vi "Defect Inspection.vi"() -> ()   [LabVIEW 2016]
doc: "Demonstrate how to use the IMAQ Calculate Defect Map function to find defects in images."
uses:
  <vilib>/vision/Pattern Matching.llb/IMAQ Pattern Match Advanced Options.ctl
  <vilib>/vision/NI_Vision_Development_Module.lvlib
panel:
  out "Thresholded Defect Map":T1(plugin-control)
  out "Defect Map":T1(plugin-control)
  out "Inspection Image":T1(plugin-control)
  out "Weight Map":T1(plugin-control)
  in  "Select Image":i32(slide) min=0 max=5 step=1 scale=0.0..4.0
  in  "Stop Button":bool
  out "Template":T1(plugin-control)
  # "Overview: Demonstrate how to use the IMAQ Calculate Defect Map function to find defects in images.\nThe VI loads a template with a pre-defined Weight Map and calls IMAQ Match Pattern 4  to find a match. IMAQ Calculate Defect Map calculates the defect map with a score for every pixel. High scores indicate a high probability for the pixels to be a defect.\nRequirements: Vision Development Module.\n\nInstructions:\n1. Run the VI.\n2. Use \"Select Image\" control to process a different image."
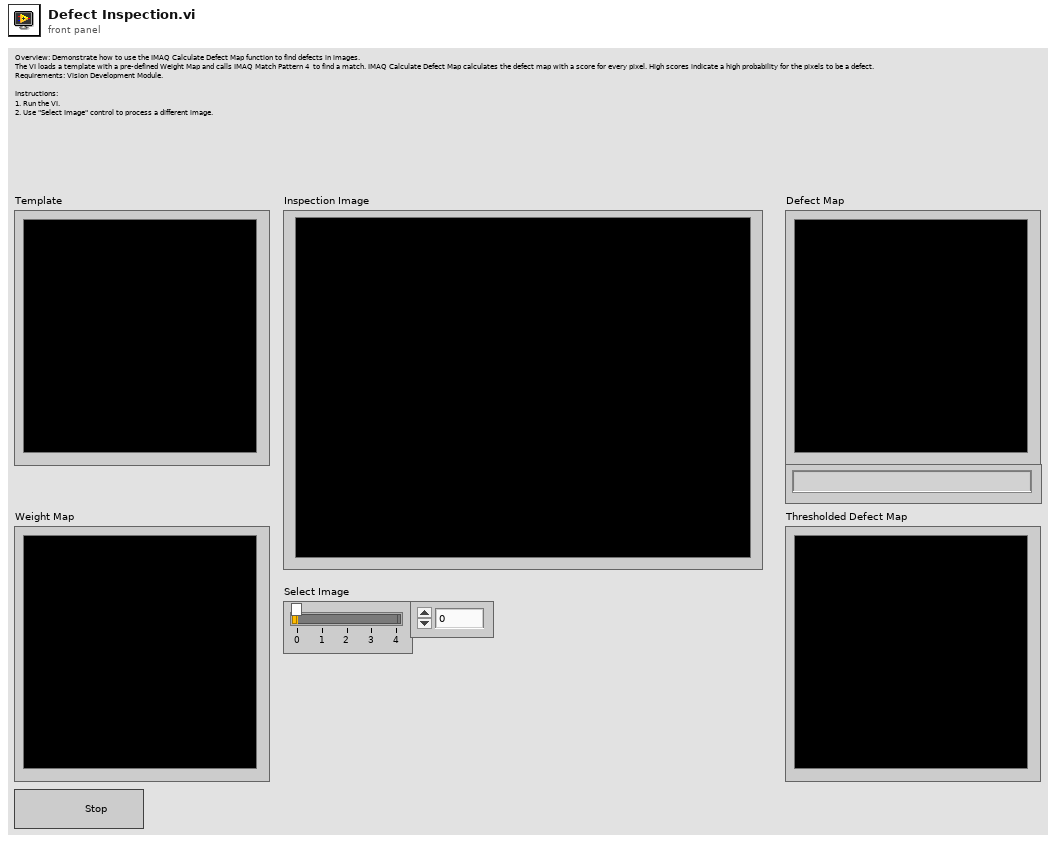
[diagram p1: front panel]
types:
  T1 = typedef "IMAQ Image.ctl" = refnum<image>
  T2 = typedef "Image Type" = u32
  T3 = typedef "IMAQ Pattern Match Advanced Options.ctl" = u16
  T4 = cluster{"Number of Matches Requested":i32, "Minimum Match Score":sgl, "Angle Ranges":cluster{"Start Angle":sgl, "End Angle":sgl}[]}
  T5 = cluster{"Position":cluster{"x":sgl, "y":sgl}, "Angle":sgl, "Scale":sgl, "Score":sgl, "Bounding Box":cluster{"x":sgl, "y":sgl}[]}[]
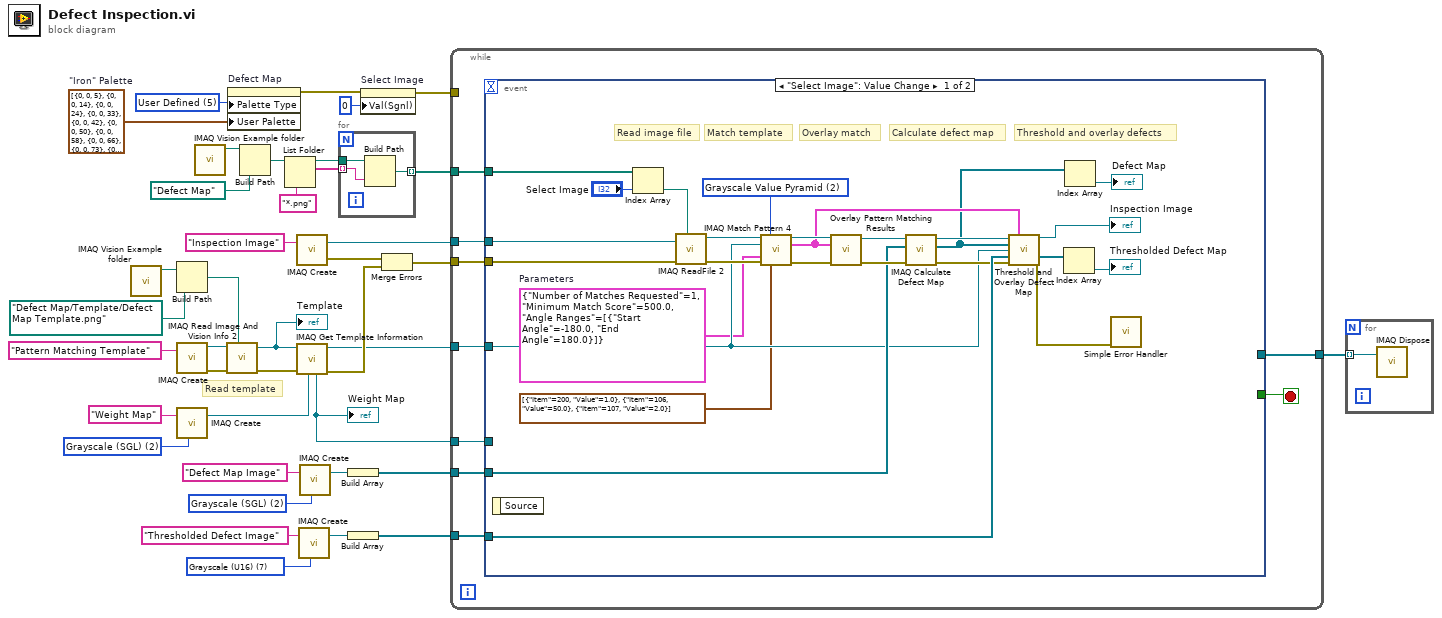
[diagram p0: block diagram]
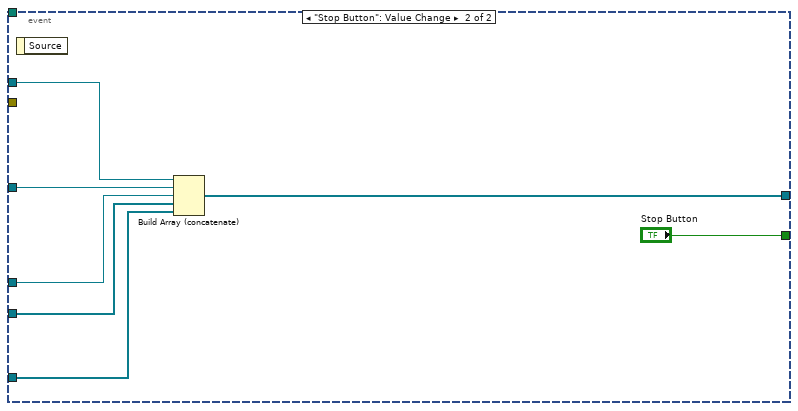
[diagram p2: hidden frame]
diagram:
  w3 = u32 5 items=["Grayscale", "Binary", "Gradient", "Rainbow", "Temperature", "User Defined", "Binary 16 Bit", "Gradient 16 Bit", "Rainbow 16 Bit", "Temperature 16 Bit", "User Defined 16 Bit"] ("Palette:Palette Type")
  w2 = cluster{"Red":u8, "Green":u8, "Blue":u8}[] [{"Red"=0, "Green"=0, "Blue"=5}, {"Red"=0, "Green"=0, "Blue"=14}, {"Red"=0, "Green"=0, "Blue"=24}, {"Red"=0, "Green"=0, "Blue"=33}, {"Red"=0, "Green"=0, "Blue"=42}, {"Red"=0, "Green"=0, "Blue"=50}, {"Red"=0, "Green"=0, "Blue"=58}, {"Red"=0, "Green"=0, "Blue"=66}, {"Red"=0, "Green"=0, "Blue"=73}, {"Red"=0, "Green"=0, "Blue"=80}, {"Red"=0, "Green"=0, "Blue"=86}, {"Red"=0, "Green"=0, "Blue"=91}, {"Red"=1, "Green"=0, "Blue"=96}, {"Red"=2, "Green"=0, "Blue"=100}, {"Red"=3, "Green"=0, "Blue"=103}, {"Red"=4, "Green"=0, "Blue"=106}, {"Red"=5, "Green"=0, "Blue"=109}, {"Red"=7, "Green"=0, "Blue"=111}, {"Red"=9, "Green"=0, "Blue"=114}, {"Red"=11, "Green"=0, "Blue"=116}, {"Red"=13, "Green"=0, "Blue"=118}, {"Red"=16, "Green"=0, "Blue"=120}, {"Red"=18, "Green"=0, "Blue"=122}, {"Red"=21, "Green"=0, "Blue"=125}, {"Red"=24, "Green"=0, "Blue"=127}, {"Red"=28, "Green"=0, "Blue"=129}, {"Red"=31, "Green"=0, "Blue"=131}, {"Red"=34, "Green"=0, "Blue"=133}, {"Red"=38, "Green"=0, "Blue"=135}, {"Red"=41, "Green"=0, "Blue"=137}, {"Red"=44, "Green"=0, "Blue"=139}, {"Red"=47, "Green"=0, "Blue"=141}, {"Red"=50, "Green"=0, "Blue"=142}, {"Red"=53, "Green"=0, "Blue"=144}, {"Red"=56, "Green"=0, "Blue"=145}, {"Red"=59, "Green"=0, "Blue"=146}, {"Red"=61, "Green"=0, "Blue"=147}, {"Red"=64, "Green"=0, "Blue"=149}, {"Red"=67, "Green"=0, "Blue"=149}, {"Red"=69, "Green"=0, "Blue"=150}, {"Red"=72, "Green"=0, "Blue"=151}, {"Red"=75, "Green"=0, "Blue"=152}, {"Red"=77, "Green"=0, "Blue"=152}, {"Red"=80, "Green"=0, "Blue"=153}, {"Red"=83, "Green"=0, "Blue"=153}, {"Red"=86, "Green"=0, "Blue"=154}, {"Red"=89, "Green"=0, "Blue"=154}, {"Red"=91, "Green"=0, "Blue"=154}, {"Red"=94, "Green"=0, "Blue"=154}, {"Red"=97, "Green"=0, "Blue"=155}, {"Red"=100, "Green"=0, "Blue"=155}, {"Red"=103, "Green"=0, "Blue"=155}, {"Red"=106, "Green"=0, "Blue"=156}, {"Red"=109, "Green"=0, "Blue"=156}, {"Red"=112, "Green"=0, "Blue"=156}, {"Red"=115, "Green"=0, "Blue"=156}, {"Red"=117, "Green"=0, "Blue"=157}, {"Red"=120, "Green"=0, "Blue"=157}, {"Red"=123, "Green"=0, "Blue"=157}, {"Red"=126, "Green"=0, "Blue"=157}, {"Red"=129, "Green"=0, "Blue"=157}, {"Red"=132, "Green"=0, "Blue"=157}, {"Red"=135, "Green"=0, "Blue"=157}, {"Red"=137, "Green"=0, "Blue"=157}, {"Red"=140, "Green"=0, "Blue"=157}, {"Red"=143, "Green"=0, "Blue"=156}, {"Red"=146, "Green"=0, "Blue"=156}, {"Red"=148, "Green"=0, "Blue"=156}, {"Red"=151, "Green"=0, "Blue"=156}, {"Red"=154, "Green"=0, "Blue"=155}, {"Red"=156, "Green"=0, "Blue"=155}, {"Red"=158, "Green"=0, "Blue"=155}, {"Red"=161, "Green"=0, "Blue"=154}, {"Red"=163, "Green"=0, "Blue"=154}, {"Red"=165, "Green"=0, "Blue"=154}, {"Red"=167, "Green"=0, "Blue"=153}, {"Red"=170, "Green"=0, "Blue"=153}, {"Red"=172, "Green"=0, "Blue"=152}, {"Red"=173, "Green"=0, "Blue"=152}, {"Red"=175, "Green"=0, "Blue"=152}, {"Red"=177, "Green"=0, "Blue"=151}, {"Red"=179, "Green"=0, "Blue"=150}, {"Red"=180, "Green"=1, "Blue"=150}, {"Red"=182, "Green"=1, "Blue"=149}, {"Red"=183, "Green"=2, "Blue"=148}, {"Red"=185, "Green"=2, "Blue"=148}, {"Red"=186, "Green"=3, "Blue"=147}, {"Red"=187, "Green"=4, "Blue"=146}, {"Red"=188, "Green"=4, "Blue"=146}, {"Red"=190, "Green"=5, "Blue"=145}, {"Red"=191, "Green"=6, "Blue"=144}, {"Red"=192, "Green"=7, "Blue"=143}, {"Red"=194, "Green"=8, "Blue"=142}, {"Red"=195, "Green"=9, "Blue"=142}, {"Red"=196, "Green"=10, "Blue"=141}, {"Red"=197, "Green"=11, "Blue"=140}, {"Red"=198, "Green"=13, "Blue"=139}, {"Red"=200, "Green"=14, "Blue"=137}, {"Red"=201, "Green"=15, "Blue"=136}, {"Red"=202, "Green"=17, "Blue"=135}, {"Red"=203, "Green"=18, "Blue"=133}, {"Red"=204, "Green"=20, "Blue"=131}, {"Red"=205, "Green"=21, "Blue"=129}, {"Red"=206, "Green"=23, "Blue"=127}, {"Red"=207, "Green"=24, "Blue"=125}, {"Red"=208, "Green"=26, "Blue"=122}, {"Red"=209, "Green"=28, "Blue"=119}, {"Red"=210, "Green"=30, "Blue"=116}, {"Red"=211, "Green"=31, "Blue"=113}, {"Red"=212, "Green"=33, "Blue"=110}, {"Red"=213, "Green"=35, "Blue"=106}, {"Red"=214, "Green"=37, "Blue"=102}, {"Red"=215, "Green"=39, "Blue"=98}, {"Red"=216, "Green"=40, "Blue"=94}, {"Red"=217, "Green"=42, "Blue"=89}, {"Red"=218, "Green"=44, "Blue"=85}, {"Red"=219, "Green"=46, "Blue"=80}, {"Red"=220, "Green"=48, "Blue"=75}, {"Red"=221, "Green"=49, "Blue"=71}, {"Red"=222, "Green"=51, "Blue"=66}, {"Red"=223, "Green"=53, "Blue"=61}, {"Red"=224, "Green"=55, "Blue"=56}, {"Red"=225, "Green"=57, "Blue"=51}, {"Red"=226, "Green"=58, "Blue"=47}, {"Red"=227, "Green"=60, "Blue"=42}, {"Red"=228, "Green"=62, "Blue"=38}, {"Red"=229, "Green"=64, "Blue"=34}, {"Red"=230, "Green"=66, "Blue"=30}, {"Red"=231, "Green"=67, "Blue"=26}, {"Red"=231, "Green"=69, "Blue"=23}, {"Red"=232, "Green"=71, "Blue"=20}, {"Red"=233, "Green"=73, "Blue"=17}, {"Red"=233, "Green"=75, "Blue"=15}, {"Red"=234, "Green"=77, "Blue"=13}, {"Red"=234, "Green"=78, "Blue"=12}, {"Red"=235, "Green"=80, "Blue"=10}, {"Red"=235, "Green"=82, "Blue"=9}, {"Red"=236, "Green"=84, "Blue"=8}, {"Red"=236, "Green"=86, "Blue"=7}, {"Red"=237, "Green"=87, "Blue"=7}, {"Red"=237, "Green"=89, "Blue"=6}, {"Red"=237, "Green"=91, "Blue"=5}, {"Red"=238, "Green"=92, "Blue"=5}, {"Red"=239, "Green"=94, "Blue"=4}, {"Red"=239, "Green"=95, "Blue"=4}, {"Red"=240, "Green"=97, "Blue"=4}, {"Red"=240, "Green"=98, "Blue"=3}, {"Red"=241, "Green"=100, "Blue"=3}, {"Red"=241, "Green"=101, "Blue"=3}, {"Red"=242, "Green"=102, "Blue"=2}, {"Red"=242, "Green"=104, "Blue"=2}, {"Red"=242, "Green"=106, "Blue"=2}, {"Red"=243, "Green"=107, "Blue"=1}, {"Red"=243, "Green"=109, "Blue"=1}, {"Red"=243, "Green"=111, "Blue"=1}, {"Red"=244, "Green"=112, "Blue"=1}, {"Red"=244, "Green"=114, "Blue"=1}, {"Red"=244, "Green"=116, "Blue"=0}, {"Red"=244, "Green"=117, "Blue"=0}, {"Red"=245, "Green"=119, "Blue"=0}, {"Red"=245, "Green"=121, "Blue"=0}, {"Red"=245, "Green"=123, "Blue"=0}, {"Red"=246, "Green"=125, "Blue"=0}, {"Red"=246, "Green"=126, "Blue"=0}, {"Red"=247, "Green"=128, "Blue"=0}, {"Red"=247, "Green"=130, "Blue"=0}, {"Red"=247, "Green"=132, "Blue"=0}, {"Red"=248, "Green"=134, "Blue"=0}, {"Red"=248, "Green"=135, "Blue"=0}, {"Red"=249, "Green"=137, "Blue"=0}, {"Red"=249, "Green"=139, "Blue"=0}, {"Red"=249, "Green"=141, "Blue"=0}, {"Red"=250, "Green"=143, "Blue"=0}, {"Red"=250, "Green"=145, "Blue"=0}, {"Red"=250, "Green"=147, "Blue"=0}, {"Red"=251, "Green"=148, "Blue"=0}, {"Red"=251, "Green"=150, "Blue"=0}, {"Red"=251, "Green"=152, "Blue"=0}, {"Red"=252, "Green"=154, "Blue"=0}, {"Red"=252, "Green"=156, "Blue"=0}, {"Red"=252, "Green"=158, "Blue"=0}, {"Red"=252, "Green"=160, "Blue"=0}, {"Red"=252, "Green"=162, "Blue"=0}, {"Red"=253, "Green"=164, "Blue"=0}, {"Red"=253, "Green"=166, "Blue"=0}, {"Red"=253, "Green"=167, "Blue"=0}, {"Red"=253, "Green"=169, "Blue"=0}, {"Red"=253, "Green"=171, "Blue"=0}, {"Red"=254, "Green"=173, "Blue"=0}, {"Red"=254, "Green"=175, "Blue"=0}, {"Red"=254, "Green"=177, "Blue"=0}, {"Red"=254, "Green"=179, "Blue"=0}, {"Red"=254, "Green"=181, "Blue"=0}, {"Red"=255, "Green"=183, "Blue"=0}, {"Red"=255, "Green"=185, "Blue"=0}, {"Red"=255, "Green"=187, "Blue"=0}, {"Red"=255, "Green"=189, "Blue"=0}, {"Red"=255, "Green"=191, "Blue"=0}, {"Red"=255, "Green"=192, "Blue"=0}, {"Red"=255, "Green"=194, "Blue"=0}, {"Red"=255, "Green"=196, "Blue"=0}, {"Red"=255, "Green"=198, "Blue"=0}, {"Red"=255, "Green"=199, "Blue"=1}, {"Red"=255, "Green"=201, "Blue"=1}, {"Red"=255, "Green"=203, "Blue"=2}, {"Red"=254, "Green"=204, "Blue"=2}, {"Red"=254, "Green"=206, "Blue"=3}, {"Red"=254, "Green"=208, "Blue"=4}, {"Red"=254, "Green"=209, "Blue"=5}, {"Red"=254, "Green"=211, "Blue"=7}, {"Red"=254, "Green"=212, "Blue"=8}, {"Red"=254, "Green"=213, "Blue"=10}, {"Red"=254, "Green"=215, "Blue"=11}, {"Red"=254, "Green"=216, "Blue"=13}, {"Red"=254, "Green"=218, "Blue"=15}, {"Red"=254, "Green"=219, "Blue"=18}, {"Red"=255, "Green"=221, "Blue"=21}, {"Red"=255, "Green"=222, "Blue"=24}, {"Red"=255, "Green"=223, "Blue"=27}, {"Red"=255, "Green"=225, "Blue"=31}, {"Red"=255, "Green"=226, "Blue"=35}, {"Red"=255, "Green"=227, "Blue"=40}, {"Red"=255, "Green"=229, "Blue"=44}, {"Red"=255, "Green"=230, "Blue"=50}, {"Red"=255, "Green"=231, "Blue"=55}, {"Red"=255, "Green"=233, "Blue"=61}, {"Red"=255, "Green"=234, "Blue"=67}, {"Red"=255, "Green"=235, "Blue"=74}, {"Red"=255, "Green"=236, "Blue"=80}, {"Red"=255, "Green"=237, "Blue"=87}, {"Red"=255, "Green"=238, "Blue"=94}, {"Red"=255, "Green"=239, "Blue"=101}, {"Red"=255, "Green"=240, "Blue"=108}, {"Red"=255, "Green"=240, "Blue"=115}, {"Red"=255, "Green"=241, "Blue"=122}, {"Red"=255, "Green"=242, "Blue"=130}, {"Red"=255, "Green"=243, "Blue"=137}, {"Red"=255, "Green"=243, "Blue"=144}, {"Red"=255, "Green"=244, "Blue"=151}, {"Red"=255, "Green"=244, "Blue"=157}, {"Red"=255, "Green"=245, "Blue"=164}, {"Red"=255, "Green"=246, "Blue"=170}, {"Red"=255, "Green"=246, "Blue"=177}, {"Red"=255, "Green"=247, "Blue"=183}, {"Red"=255, "Green"=248, "Blue"=189}, {"Red"=255, "Green"=248, "Blue"=195}, {"Red"=255, "Green"=249, "Blue"=200}, {"Red"=255, "Green"=250, "Blue"=206}, {"Red"=255, "Green"=251, "Blue"=212}, {"Red"=255, "Green"=251, "Blue"=217}, {"Red"=255, "Green"=252, "Blue"=223}, {"Red"=255, "Green"=253, "Blue"=229}, {"Red"=255, "Green"=253, "Blue"=234}, {"Red"=255, "Green"=254, "Blue"=240}, {"Red"=255, "Green"=255, "Blue"=246}, {"Red"=255, "Green"=255, "Blue"=251}]  # "Iron" Palette
  w11 = T2 7 items=["Grayscale (U8)", "Grayscale (I16)", "Grayscale (SGL)", "Complex (CSG)", "RGB (U32)", "HSL (U32)", "RGB (U64)", "Grayscale (U16)"] ("Image Type")
  w21 = T2 2 items=["Grayscale (U8)", "Grayscale (I16)", "Grayscale (SGL)", "Complex (CSG)", "RGB (U32)", "HSL (U32)", "RGB (U64)", "Grayscale (U16)"] ("Image Type")
  w29 = T2 2 items=["Grayscale (U8)", "Grayscale (I16)", "Grayscale (SGL)", "Complex (CSG)", "RGB (U32)", "HSL (U32)", "RGB (U64)", "Grayscale (U16)"] ("Image Type")
  # "Read template"
  n1 = call "IMAQ Vision Example folder.vi"() -> ("Example Image Path"=w36:path)  [unwired: 11 in]
  n2 = Build Path(base path=w36, name or relative path=path "Defect Map/Template/Defect Map Template.png") -> (appended path=w33:path)
  n3 = call "IMAQ Create"("Image Name"="Pattern Matching Template") -> ("New Image"=w34:T1, "error out"=w27:errorcluster)  [unwired: 4 in]
  n4 = call "IMAQ Create"("Image Name"="Weight Map", "Image Type"=w29) -> ("New Image"=w28:T1)  [unwired: 3 in, 1 out]
  n5 = call "IMAQ Vision Example folder.vi"() -> ("Example Image Path"=w37:path)  [unwired: 11 in]
  n6 = call "IMAQ Read Image And Vision Info 2"("File Path"=w33, "error in (no error)"=w27, "Image"=w34) -> ("error out"=w31:errorcluster, "Image Out"=w32:T1)  [unwired: 6 in, 1 out]
  "Template" <- w32
  n7 = property on="Defect Map" class="ImageControl"("Palette Type"=w3, "User Palette"=w2) -> (error out=w1:errorcluster)  [unwired: 2 in, 1 out]
  n8 = Build Path(base path=w37, name or relative path=path "Defect Map" ("path out")) -> (appended path=w17:path)
  n9 = List Folder(path=w17, pattern="*.png") -> (path out=w15:path, filenames=w14:string[])  [unwired: 1 in, 3 out]
  n10 = call "IMAQ Create"("Image Name"="Inspection Image") -> ("New Image"=w6:T1, "error out"=w25:errorcluster)  [unwired: 4 in]
  n11 = call "IMAQ Get Template Information"("Weight Map"=w28, "error in (no error)"=w31, "Template Image"=w32) -> ("error out"=w26:errorcluster, "Template Image (duplicate)"=w7:T1, "Weight Map Out"=w5:T1)  [unwired: 3 in, 3 out]
  "Weight Map" <- w5
  n12 = call "IMAQ Create"("Image Name"="Thresholded Defect Image", "Image Type"=w11) -> ("New Image"=w10:T1)  [unwired: 3 in, 1 out]
  n13 = call "IMAQ Create"("Image Name"="Defect Map Image", "Image Type"=w21) -> ("New Image"=w22:T1)  [unwired: 3 in, 1 out]
  n14 = for {
    tunnel: w15 -> [w42]
    tunnel: w14 -> [w41] mode=indexing
    tunnel: [w40] -> w13 mode=indexing
    n15 = Build Path(base path=w42, name or relative path=w41) -> (appended path=w40:path)
  }
  n16 = Build Array(w22) -> (w8:T1[])
  n17 = Build Array(w10) -> (w9:T1[])
  n18 = property on="Select Image" class="Slide (strict)"(error in=w1, "Val(Sgnl)"=0 ("Value (Signaling)")) -> (error out=w18:errorcluster)  [unwired: 1 in, 1 out]
  n19 = Merge Errors(w25, w26) -> (w24:errorcluster)
  n20 = while {
    tunnel: w6 -> [w51]
    tunnel: w7 -> [w50]
    tunnel: w24 -> [w49]
    tunnel: w8 -> [w48]
    tunnel: w18 -> [_]
    tunnel: w13 -> [w47]
    tunnel: w9 -> [w46]
    tunnel: w5 -> [w45]
    tunnel: [w44] -> w4
    stop <- w43 stop-if-true
    n21 = event shown="[0] \"Select Image\": Value Change" {
      selector: _ -> [_ _]
      dyn-events: _ -> [_ _]
      timeout: _ -> [_ _]
      tunnel: w51 -> [w77 w79]
      tunnel: [_ "Stop Button"] -> w43
      tunnel: w50 -> [w56 w80]
      tunnel: w49 -> [w71 _]
      tunnel: w48 -> [w63 w82]
      tunnel: w47 -> [w62 _]
      tunnel: w46 -> [w59 w83]
      tunnel: w45 -> [_ w81]
      tunnel: [_ w78] -> w44
      event "Select Image": Value Change {
        w53 = 2 items=["All", "Low Discrepancy Sampling", "Grayscale Value Pyramid", "Gradients Pyramid"] ("Algorithm")
        w54 = T4 {"Number of Matches Requested"=1, "Minimum Match Score"=500.0, "Angle Ranges"=[{"Start Angle"=-180.0, "End Angle"=180.0}]}  # Parameters
        # "Threshold and overlay defects"
        # "Calculate defect map"
        # "Overlay match"
        # "Match template"
        # "Read image file"
        n22 = event-data() -> ()  [unwired: 1 in, 1 out]
        n23 = Index Array(array=w62, index="Select Image") -> (element=w61:path)
        n24 = call "IMAQ ReadFile 2"("File Path"=w61, "error in (no error)"=w71, "Image"=w77) -> ("error out"=w73:errorcluster, "Image Out"=w69:T1)  [unwired: 4 in, 3 out]
        n25 = call "IMAQ Match Pattern 4"("Image"=w69, "Algorithm"=w53, "Template Image"=w56, "Parameters"=w54, "error in (no error)"=w73, "Advanced Options"=cluster{"Item":T3, "Value":dbl}[] [{"Item"=200, "Value"=1.0}, {"Item"=106, "Value"=50.0}, {"Item"=107, "Value"=2.0}]) -> ("Image (duplicate)"=w75:T1, "Matches (pixel)"=w68:T5, "error out"=w74:errorcluster)  [unwired: 5 in, 2 out]
        n26 = call "Overlay Pattern Matching Results.vi"("error in"=w74, "Matches"=w68, "Image"=w75) -> ("error out"=w72:errorcluster, "Image Out"=w70:T1)  [unwired: 7 in]
        n27 = call "IMAQ Calculate Defect Map"("error in (no error)"=w72, "Defect Images In"=w63, "Image"=w70) -> ("error out"=w58:errorcluster, "Defect Images Out"=w55:T1[], "Image (duplicate)"=w60:T1)  [unwired: 6 in]
        n28 = call "Threshold and Overlay Defect Map.vi"("Match Image"=w60, "Matches"=w68, "Defect Images"=w55, "Template image"=w56, "Thresholded Image In"=w59, "error in"=w58) -> ("Match Image Out"=→"Inspection Image":T1, "Thresholded Image Out"=w67:T1[], "error out"=w57:errorcluster)  [unwired: 7 in]
        n29 = Index Array(array=w67) -> (element=→"Thresholded Defect Map":T1)  [unwired: 1 in]
        n30 = Index Array(array=w55) -> (element=→"Defect Map":T1)  [unwired: 1 in]
        n31 = call <vilib>:"Simple Error Handler.vi"("error in (no error)"=w57) -> ()  [unwired: 4 in, 5 out]
      }
      event "Stop Button": Value Change {
        n32 = event-data() -> ()  [unwired: 1 in, 1 out]
        n33 = Build Array (concatenate)(w79, w80, w81, w82, w83) -> (w78:T1[])
      }
    }
  }
  n34 = for {
    tunnel: w4 -> [w85] mode=indexing
    n35 = call "IMAQ Dispose"("Image"=w85) -> ()  [unwired: 5 in, 1 out]
  }
